vi "Passive Force Clamp-final.vi"(4 "file name add to the end (height)":string="h300", 5 "feedback?":bool, 6 "X=T,Y=F":bool=TRUE, 7 "save?":bool, 8 "Intensity Control, 0~-7000 (mV)":dbl=-1200.0 format="%_8g", 9 "moving step size (um)":dbl=0.05, 10 "upper set value":dbl=0.34, 11 "range (um)":dbl=2.0 format="%.3f") -> ()   [LabVIEW 2014]
uses:
  <vilib>/Analysis/baseanly.llb/Mean (DBL).vi
  Main-Stage-Based/(Global) Current handle and LaserPower_YCC.vi
  <vilib>/Analysis/NI_AALBase.lvlib
panel:
  out "target QPD (V)":dbl
  in  "Avg. time delay (ms)":dbl=20.0
  out "True Target position":dbl
  in  "averged delay":dbl=18.0
  out "Record scan rate  (um/s)":dbl=2.0
  out "Laser Lock?":bool
  out "Center QPD yc (V)":dbl format="%0.2f"
  out "Sampling rate after filtering (Hz)":dbl
  in  "Who's Data":enum16{"YCC", "PYW", "LCH", "YYH"}(ring)
  in  "left rank":i32=160
  out "Stage-QPD data":dbl[][](array[numeric])
  out "Now position (um)":dbl
  in  "Avg points":i32=320
  out "True rate?":bool
  out "Real initial position (um)":dbl format="%0.5f"
  out "Axis":i32
  in  "toward+ ?\nT=+, F=-":bool
  out "target position (um)":dbl
  in  "extension = T\ncontraction = F":bool=TRUE
  in  "stop":bool
  in  "Tab Control":enum32{"Stage movment", "Raw Data", "All Data"}(tab)
  out "XY Graph":T1(graph)
  in  "Set Target position?":bool
  out "Z-QPD":dbl(graph)
  out "Waveform Chart":dbl[](graph)
  out "XY Graph 2":cluster{dbl[], "Filtered X":dbl[]}[](graph)
  in  "Sampling rate":dbl=32000.0
  # "2.9um for had acted"
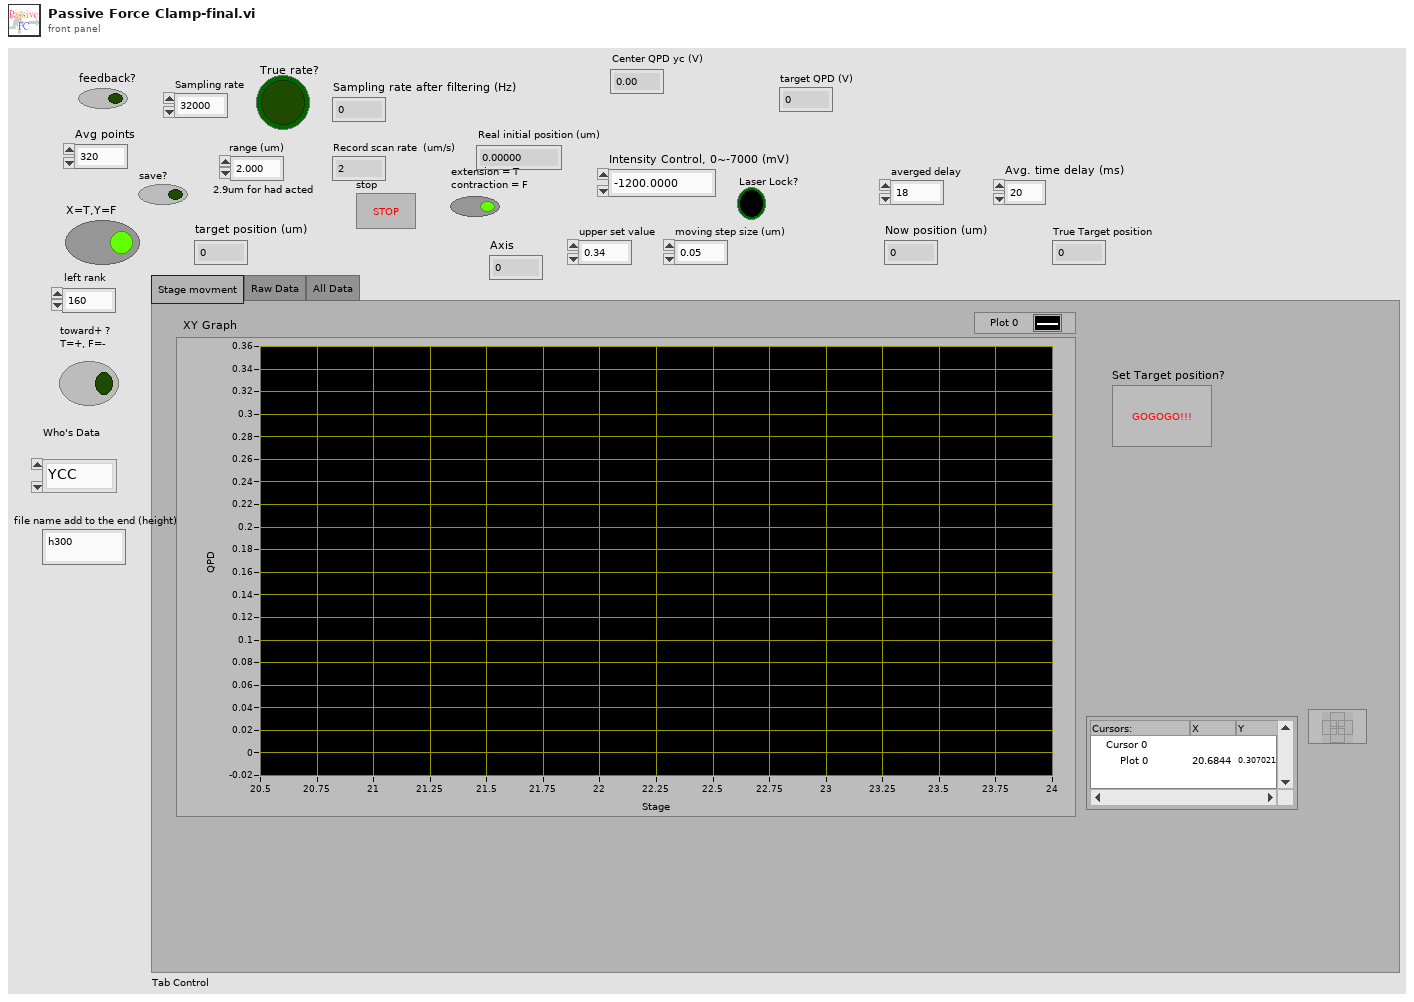
[diagram p1: front panel]
types:
  T1 = cluster{"Filtered Stage Array":dbl[], "Filtered QPD data":dbl[]}
  T2 = enum16{"Fixed-window avg", "Moving-window avg", "F+S-window avg", "S-G filter", "Fixed-window Median", "Moving-window Median "}
  T3 = cluster{"Correct Unfolded Stage Array (um)":dbl[], "Filtered QPD Array":dbl[]}
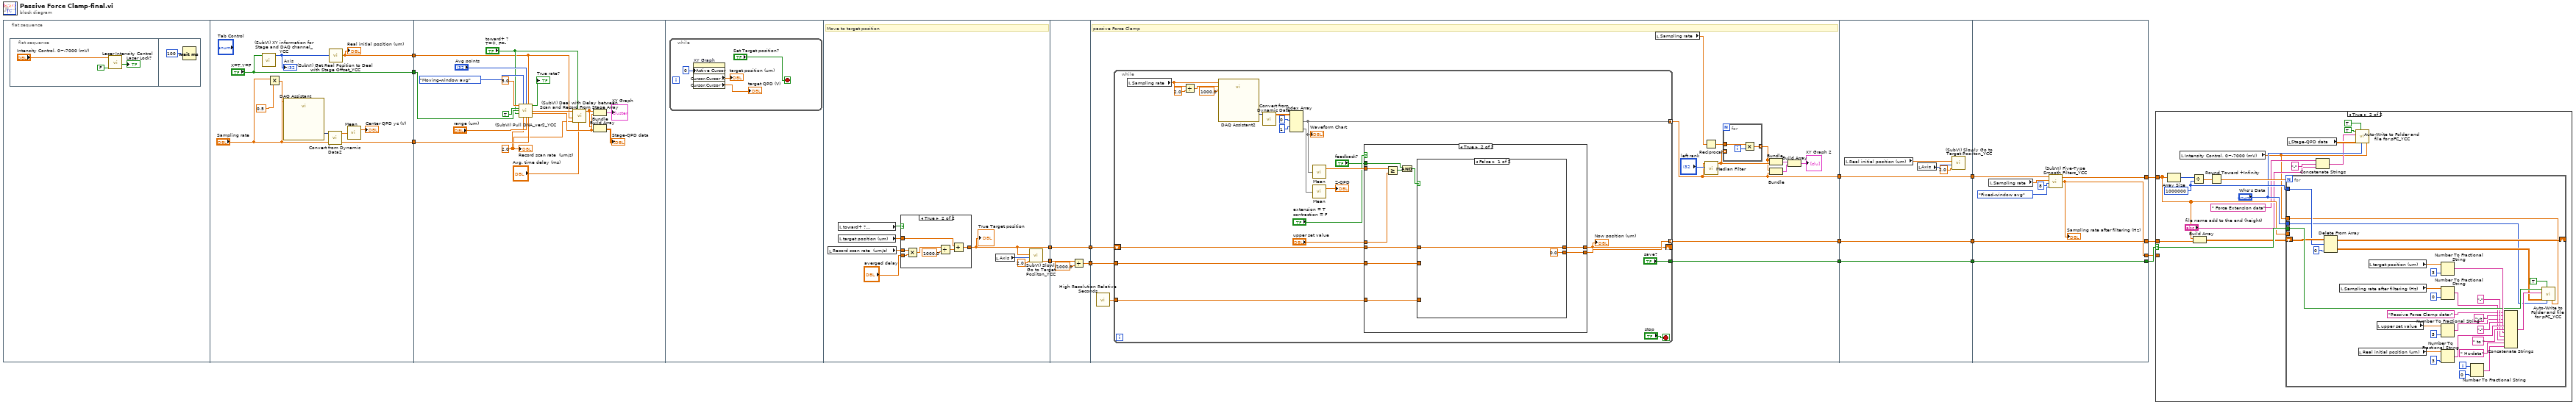
[diagram p0: block diagram]
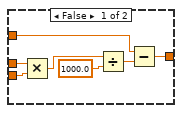
[diagram p3: hidden frame]
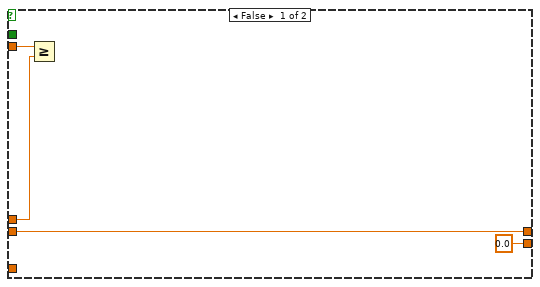
[diagram p4: hidden frame]
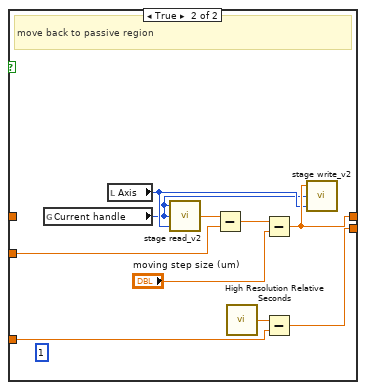
[diagram p5: hidden frame]
diagram:
  n1 = flat-sequence {
    tunnel: [w29] -> w14
    tunnel: ["X=T,Y=F"] -> w13
    tunnel: ["Sampling rate"] -> w2
    tunnel: w14 -> [w34]
    tunnel: w13 -> [w39]
    tunnel: w2 -> [w38]
    tunnel: [w52] -> w12
    tunnel: [w57] -> w1
    tunnel: w12 -> [w77]
    tunnel: [w77] -> w11
    tunnel: [w75] -> w10
    tunnel: w1 -> [w74]
    tunnel: w11 -> [w88]
    tunnel: w10 -> [w87]
    tunnel: [w81] -> w8
    tunnel: [w90] -> w6
    tunnel: [w89] -> w4
    tunnel: w8 -> [w148]
    tunnel: [w148] -> w7
    tunnel: w6 -> [w147]
    tunnel: [w147] -> w5
    tunnel: w4 -> [w146]
    tunnel: [w146] -> w3
    tunnel: [w155] -> w15
    tunnel: [w156] -> w16
    tunnel: [w150] -> w17
    tunnel: w7 -> [w154]
    tunnel: w5 -> [w156]
    tunnel: w3 -> [w155]
    tunnel: [w151] -> w9
    frame #0 {
      n2 = flat-sequence {
        frame #0 {
          n3 = call "Laser Intensity Control.vi"("Close?"=FALSE, "Intensity Control, 0~-7000 (mV)"="Intensity Control, 0~-7000 (mV)") -> ("Laser Lock?"=→"Laser Lock?":bool)  [unwired: 5 in]
        }
        frame #1 {
          n4 = Wait (ms)(milliseconds to wait=u32 100) -> ()  [unwired: 1 out]
        }
      }
    }
    frame #1 {
      n5 = call "(SubVI) XY information for Stage and DAQ channel_YCC.vi"("T=X\nF=Y"="X=T,Y=F") -> ("Axis"=w30:i32)  [unwired: 3 in, 1 out]
      "Axis" <- w30
      n6 = Multiply(x="Sampling rate", y=0.5) -> (x*y=w25:dbl)
      n7 = call "DAQ Assistant"("rate"="Sampling rate", "number of samples"=w25) -> ("data"=w24:dynamicdata)  [unwired: 15 in, 2 out]
      n8 = call "Convert from Dynamic Data2"("Dynamic Data Type"=w24) -> ("Array"=w23:dbl[])  [unwired: 3 in]
      n9 = call "(SubVI) Get Real Position to Deal with Stage Offset_YCC.vi"("Axis"=w30) -> ("Real Current Commanded position (um)"=w29:dbl)  [unwired: 3 in, 1 out]
      "Real initial position (um)" <- w29
      n10 = call-poly <vilib>:"Mean.vi"("X"=w23) -> ("mean"=→"Center QPD yc (V)":dbl)  [unwired: 1 out]
    }
    frame #2 {
      w33 = 2.0 ("Record scan rate  (um/s)")
      n11 = call "(SubVI) Pull DNA_ver2_YCC.vi"("waiting time per point (ms)\nrange from 5ms to 0.167 ms"=5.0 ("waiting time per point (ms)\nrange from 5ms to 0.167 ms"), "Filter type"=T2."Moving-window avg", "Avg points"="Avg points", "Real initial position (um)"=w34, "Record?"=TRUE, "T=X\nF=Y"=w39, "Toward  ?\nT=+, F=-"="toward+ ?\nT=+, F=-", "Record scan rate  (um/s)"=w33, "range  (um)"="range (um)", "Sampling rate"=w38) -> ("True rate?"=→"True rate?":bool, "Filtered Stage Array"=w36:dbl[], "Filtered QPD Array"=w47:dbl[])  [unwired: 2 in, 1 out]
      n12 = call "(SubVI) Deal with Delay between Scan and Record From Stage Array.vi"("Avg. time delay (ms)"="Avg. time delay (ms)", "Toward first ?\nT=+, F=-"="toward+ ?\nT=+, F=-", "Record scan rate  (um/s)"=w33, "Real initial position (um)"=w34, "Unfolded Stage Array (um)"=w36) -> ("Correct Unfolded Stage Array (um)"=w31:dbl[])  [unwired: 2 in, 2 out]
      n13 = Bundle("Correct Unfolded Stage Array (um)"=w31, "Filtered QPD Array"=w47) -> (→"XY Graph":T3)  [unwired: 1 in]
      n14 = Build Array(w31, w47) -> (→"Stage-QPD data":dbl[][])
      "Record scan rate  (um/s)" <- w33
    }
    frame #3 {
      n15 = while {
        stop <- "Set Target position?" stop-if-true
        n16 = property on="XY Graph" class="XYGraph (strict)"("Active Cursor"=u32 0) -> ("Cursor.Cursor X"=→"target position (um)":dbl, "Cursor.Cursor Y"=→"target QPD (V)":dbl)  [unwired: 2 in, 2 out]
      }
    }
    frame #4 {
      # "Move to target position"
      n17 = local read "Record scan rate  (um/s)"() -> (w53:dbl)
      n18 = local read "toward+ ?\nT=+, F=-"() -> (w55:bool)
      n19 = local read "target position (um)"() -> (w56:dbl)
      n20 = case shown="True" w55 {
        tunnel: w56 -> [w66 w69]
        tunnel: [w62 w67] -> w52
        tunnel: "averged delay" -> [w61 w70]
        tunnel: w53 -> [w60 w71]
        frame False {
          n21 = Multiply(x=w60, y=w61) -> (x*y=w65:dbl)
          n22 = Divide(x=w65, y=1000.0) -> (x/y=w63:dbl)
          n23 = Subtract(x=w66, y=w63) -> (x-y=w62:dbl)
        }
        frame True {
          n24 = Multiply(x=w71, y=w70) -> (x*y=w73:dbl)
          n25 = Divide(x=w73, y=1000.0) -> (x/y=w68:dbl)
          n26 = Add(x=w69, y=w68) -> (x+y=w67:dbl)
        }
      }
      "True Target position" <- w52
      n27 = local read "Axis"() -> (w59:i32)
      n28 = call "(SubVI) Slowly Go to Target Posiiton_YCC.vi"("scan rate  (um/s)"=2.0, "axis"=w59, "Target position (um)"=w52) -> ("Expect - Real move (nm)\nStage Offset\n+=more move\n-=less move"=w57:dbl)  [unwired: 1 in, 3 out]
    }
    frame #5 {
      n29 = Divide(x=w74, y=1000.0) -> (x/y=w75:dbl)
    }
    frame #6 {
      # "passive Force Clamp"
      n30 = call <vilib>:"High Resolution Relative Seconds.vi"() -> ("relative seconds"=w91:dbl)
      n31 = while {
        tunnel: w91 -> [w112]
        tunnel: [w111] -> w90 mode=indexing
        tunnel: [w97] -> w81 mode=concatenating
        tunnel: ["save?"] -> w89
        shift-right: [w101] -> _
        shift-left: w88 -> [w102]
        tunnel: w87 -> [w103]
        stop <- "stop" stop-if-true
        n32 = local read "Sampling rate"() -> (w106:dbl)
        n33 = Divide(x=w106, y=2.0) -> (x/y=w104:dbl)
        n34 = call "DAQ Assistant2"("rate"=w106, "number of samples"=w104, "timeout (s)"=1000.0) -> ("data"=w109:dynamicdata)  [unwired: 13 in, 3 out]
        n35 = call "Convert from Dynamic Data"("Dynamic Data Type"=w109) -> ("Array"=w100:dbl[][])  [unwired: 3 in]
        n36 = Index Array(array=w100, index (row) #1=0 ("index (row)"), index (row) #2=1 ("index (row)")) -> (element #1=w97:dbl[], element #2=w96:dbl[])  [unwired: 2 in]
        "Waveform Chart" <- w97
        n37 = call-poly <vilib>:"Mean.vi"("X"=w97) -> ("mean"=w115:dbl)  [unwired: 1 out]
        n38 = call-poly <vilib>:"Mean.vi"("X"=w96) -> ("mean"=→"Z-QPD":dbl)  [unwired: 1 out]
        n39 = case shown="True" "extension = T\ncontraction = F" {
          tunnel: w115 -> [w120 w130]
          tunnel: "upper set value" -> [w119 w129]
          tunnel: w112 -> [_ w128]
          tunnel: [0.0 w127] -> w111
          tunnel: [w117 w124] -> w101
          tunnel: "feedback?" -> [_ w123]
          tunnel: w103 -> [_ w122]
          tunnel: w102 -> [w117 w121]
          frame False {
            n40 = Greater Or Equal?(x=w120, y=w119) -> ()  [unwired: 1 out]
          }
          frame True {
            n41 = Greater Or Equal?(x=w130, y=w129) -> (x >= y?=w126:bool)
            n42 = And(x=w123, y=w126) -> (x .and. y?=w125:bool)
            n43 = case shown="False" w125 {
              tunnel: w128 -> [_ w141]
              tunnel: [0.0 w139] -> w127
              tunnel: [w131 w138] -> w124
              tunnel: w122 -> [_ w135]
              tunnel: w121 -> [w131 _]
              frame False {
              }
              frame True {
                (unwired) 1 ("read #")
                # "move back to passive region"
                n44 = global read "(Global) Current handle and LaserPower_YCC.vi" "Current handle"() -> (w133:i32)
                n45 = local read "Axis"() -> (w137:i32)
                n46 = call "stage read_v2.vi"("Axis"=w137, "Incoming Handle"=w133, "read #"=w133) -> ("position (um)"=w136:dbl)  [unwired: 1 in, 1 out]
                n47 = Subtract(x=w136, y=w135) -> (x-y=w134:dbl)
                n48 = call <vilib>:"High Resolution Relative Seconds.vi"() -> ("relative seconds"=w140:dbl)
                n49 = Subtract(x=w134, y="moving step size (um)") -> (x-y=w138:dbl)
                n50 = Subtract(x=w140, y=w141) -> (x-y=w139:dbl)
                n51 = call "stage write_v2.vi"("axis"=w137, "Incoming Handle"=w133, "position"=w138) -> ()  [unwired: 2 in, 1 out]
              }
            }
          }
        }
        "Now position (um)" <- w101
      }
      n52 = local read "Sampling rate"() -> (w85:dbl)
      n53 = Reciprocal(x=w85) -> (1/x=w84:dbl)
      n54 = call <vilib>:"Median Filter.vi"("left rank"="left rank", "X"=w81) -> ("Filtered X"=w83:dbl[])  [unwired: 8 in, 1 out]
      n55 = for {
        tunnel: w83 -> [_] mode=indexing
        tunnel: w84 -> [w93]
        tunnel: [w92] -> w82 mode=indexing
        i -> [w94]
        n56 = Multiply(x=w93, y=w94) -> (x*y=w92:dbl)
      }
      n57 = Bundle(w82, "Filtered X"=w83) -> (w79:cluster{dbl[], "Filtered X":dbl[]})  [unwired: 1 in]
      n58 = Bundle(w82, "Array"=w81) -> (w78:cluster{dbl[], "Array":dbl[]})  [unwired: 1 in]
      n59 = Build Array(w79, w78) -> (→"XY Graph 2":cluster{dbl[], "Array":dbl[]}[])
    }
    frame #7 {
      n60 = local read "Real initial position (um)"() -> (w144:dbl)
      n61 = local read "Axis"() -> (w145:i32)
      n62 = call "(SubVI) Slowly Go to Target Posiiton_YCC.vi"("scan rate  (um/s)"=2.0, "axis"=w145, "Target position (um)"=w144) -> ()  [unwired: 1 in, 4 out]
    }
    frame #8 {
      n63 = local read "Sampling rate"() -> (w153:dbl)
      n64 = call "(SubVI) Five-Type Smooth Filters_YCC.vi"("Filter type"=T2."Fixed-window avg", "Avg points"=8, "Sampling rate (Hz)"=w153, "QPD data"=w154) -> ("Sampling rate after filtering (Hz)"=w151:dbl, "Filtered QPD data"=w150:dbl[])  [unwired: 1 in]
      "Sampling rate after filtering (Hz)" <- w151
    }
  }
  n65 = case shown="True" w15 {
    selector: w15 -> [_ w173]
    tunnel: w17 -> [_ w169]
    tunnel: w16 -> [_ w168]
    tunnel: w9 -> [_ _]
    frame False {
    }
    frame True {
      w166 = 1000000 ("y")
      n66 = Array Size(array=w169) -> (size(s)=w170:i32)
      n67 = local read "Intensity Control, 0~-7000 (mV)"() -> (w157:dbl)
      n68 = Divide(x=w170, y=w166) -> (x/y=w172:dbl)
      n69 = Build Array(w169, w168) -> (w167:dbl[][])
      n70 = Round Toward +Infinity(x=w172) -> (ceil(x): smallest int >= x=w171:dbl)
      n71 = for {
        N: w171 -> [_]
        tunnel: w169 -> [_]
        tunnel: w173 -> [w195]
        shift-right: [w181] -> _
        shift-left: w167 -> [w186]
        tunnel: w166 -> [w185]
        tunnel: "Who's Data" -> [w180]
        tunnel: w157 -> [w174]
        i -> [w193]
        n72 = Delete From Array(array=w186, length=w185, index (col)=0 ("index (row)")) -> (deleted portion=w183:dbl[][], array with subset deleted=w181:dbl[][])  [unwired: 1 in]
        n73 = local read "Sampling rate after filtering (Hz)"() -> (w194:dbl)
        n74 = local read "Real initial position (um)"() -> (w204:dbl)
        n75 = local read "target position (um)"() -> (w201:dbl)
        n76 = local read "upper set value"() -> (w177:dbl)
        n77 = Number To Fractional String(number=w201, precision (6)=i16 3) -> (F-format string=w198:string)  [unwired: 2 in]
        n78 = Number To Fractional String(number=w194, precision (6)=i16 0) -> (F-format string=w189:string)  [unwired: 2 in]
        n79 = Number To Fractional String(number=w177, precision (6)=i16 5) -> (F-format string=w175:string)  [unwired: 2 in]
        n80 = Number To Fractional String(number=w204, precision (6)=i16 3) -> (F-format string=w200:string)  [unwired: 2 in]
        n81 = Number To Fractional String(number=w193, precision (6)=i16 0) -> (F-format string=w187:string)  [unwired: 2 in]
        n82 = Concatenate Strings("Passive Force Clamp data-" ("prompt"), "yt " ("string"), w175, "-" ("string"), w200, " to " ("string"), w198, "-" ("string"), w189, " Hz-data" ("string"), w187) -> (w196:string)
        n83 = call "Auto-Write to Folder and file for pFC_YCC.vi"("Current PD (mV)"=w174, "Who's Data"=w180, "T=2D\nF=1D"=TRUE ("T=2D\nF=1D"), "2D data to be saved"=w183, "File name add to the end \n(height)"=w196, "Save?"=w195) -> ()  [unwired: 2 in, 2 out]
      }
      n84 = local read "Stage-QPD data"() -> (w165:dbl[][])
      n85 = Concatenate Strings(" Force Extension data" ("prompt"), "-" ("string"), "file name add to the end (height)") -> (w158:string)
      n86 = call "Auto-Write to Folder and file for pFC_YCC.vi"("Current PD (mV)"=w157, "Who's Data"="Who's Data", "T=2D\nF=1D"=TRUE ("T=2D\nF=1D"), "2D data to be saved"=w165, "File name add to the end \n(height)"=w158, "Save?"=TRUE) -> ()  [unwired: 2 in, 2 out]
    }
  }
